vi "Get Property Values (Path Property).vi"(1 "data type":path[](array[path]), 5 "property":T2 {"data type" items=["Unknown"=0, "String"=23, "I32"=3, "I64"=4, "DBL"=10, "Time stamp"=30]; "object type" items=["File", "Channel Group", "Channel"]}, 7 "result references":T1[](array[typedef]), 11 "error in (no error)":errorcluster) -> (6 "property values":path[](array[path]), 8 "result references out":T1[](array[typedef]), 15 "error out":errorcluster)   [LabVIEW 2020, in "NI_DataFinder.lvlib"]
doc: "Determines from the result references the values of a path property."
uses:
  <vilib>/DataFinder/NI_DataFinder.lvlib
  <vilib>/DataFinder/DataTypes/property.ctl
  <vilib>/DataFinder/DataTypes/object type.ctl
  <vilib>/DataFinder/DataTypes/data type.ctl
  <vilib>/userdefined/DFSearchResult.ctl
  <vilib>/userdefined/NI_DataFinder Controls.lvlib
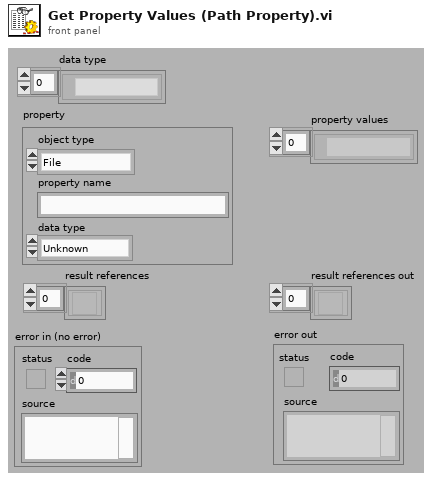
[diagram p1: front panel]
types:
  T1 = typedef "NI_DataFinder Controls.lvlib/DFSearchResult.ctl" = refnum<k20>
  T2 = typedef "NI_DataFinder.lvlib/property.ctl" = cluster{"object type":T3, "property name":string, "data type":T4}
  T3 = typedef "NI_DataFinder.lvlib/object type.ctl" = u16
  T4 = typedef "NI_DataFinder.lvlib/data type.ctl" = u16
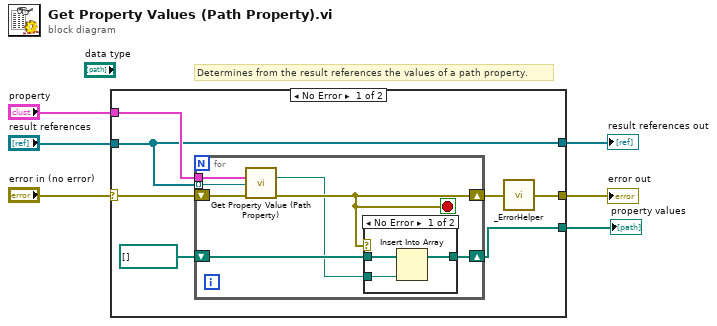
[diagram p0: block diagram]
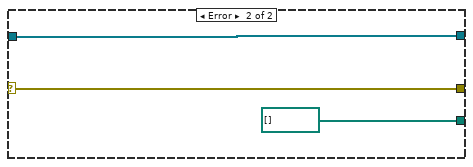
[diagram p3: hidden frame]
diagram:
  # "Determines from the result references the values of a path property."
  n1 = case shown="No Error" "error in (no error)" {
    selector: "error in (no error)" -> [w13 w27]
    tunnel: [w11 w27] -> w5
    tunnel: [w10 w26] -> w1
    tunnel: [w7 path[] []] -> w3
    tunnel: "result references" -> [w10 w26]
    tunnel: "property" -> [w12 _]
    frame No Error {
      n2 = for {
        tunnel: w10 -> [w17] mode=indexing
        tunnel: w12 -> [w16]
        shift-right: [w15] -> w9
        shift-left: w13 -> [w18]
        shift-right: [w19] -> w7
        shift-left: path[] [] ("property values") -> [w20]
        stop <- w15 stop-if-true
        n3 = call <vilib>:"Get Property Value (Path Property).vi"("property"=w16, "result reference"=w17, "error in (no error)"=w18) -> ("property value"=w14:path, "error out"=w15:errorcluster)  [unwired: 10 in, 1 out]
        n4 = case shown="No Error" w15 {
          tunnel: w20 -> [w22 w24]
          tunnel: [w23 w24] -> w19
          tunnel: w14 -> [w21 _]
          frame No Error {
            n5 = Insert Into Array(array=w22, new element=w21) -> (w23:path[])  [unwired: 1 in]
          }
          frame Error {
          }
        }
      }
      n6 = call <vilib>:"_ErrorHelper.vi"("error IO"=w9) -> ("error out"=w11:errorcluster)
    }
    frame Error {
    }
  }
  "property values" <- w3
  "error out" <- w5
  "result references out" <- w1
